vi "NATS Request.vi"(0 "nats connection in":T3={"connection ID"=refnum, "server INFO"="", "timeout ms"=5000, "verbose?"=FALSE, "server headers?"=FALSE, "client headers?"=FALSE}, 1 "reply-to":string, 2 "request queue":refnum<queue>, 5 "subject":string, 7 "payload":string, 9 "sub id":string, 11 "error in":errorcluster, 12 "timeout ms (conn default)":i32=-2, 13 "bytes to read (1024)":i32=1024) -> (4 "nats message":T1, 15 "error out":errorcluster)   [LabVIEW 2023, in "NATS Core.lvlib"]
doc: "Publishes a message to the NATS server."
uses:
  NATS Core.lvlib
  Controls/nats connection.ctl
  <vilib>/dlg_ctls.llb/Space Constant.vi
  subVIs/Set Timeout.vi
  Controls/msg type.ctl
  Controls/nats message.ctl
  Controls/request queue.ctl
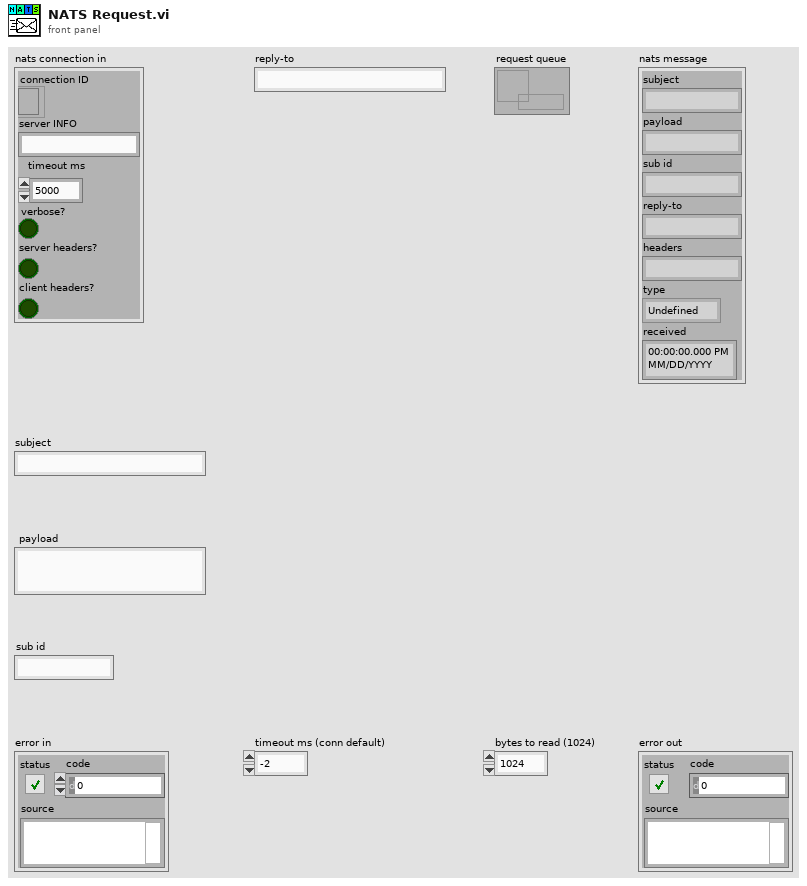
[diagram p1: front panel]
types:
  T1 = typedef "NATS Core.lvlib/nats message.ctl" = cluster{"subject":string, "payload":string, "sub id":string, "reply-to":string, "headers":string, "type":T2, "received":timestamp}
  T2 = typedef "NATS Core.lvlib/msg type.ctl" = enum16{"Undefined", "MSG", "HMSG", "+OK", "PING", "PONG", "-ERR", "INFO"}
  T3 = typedef "NATS Core.lvlib/nats connection.ctl" = cluster{"connection ID":refnum<k5>, "server INFO":string, "timeout ms":i32, "verbose?":bool, "server headers?":bool, "client headers?":bool}
  T4 = typedef "request queue.ctl" = cluster{"reply subject":string, "request queue":refnum<queue>}
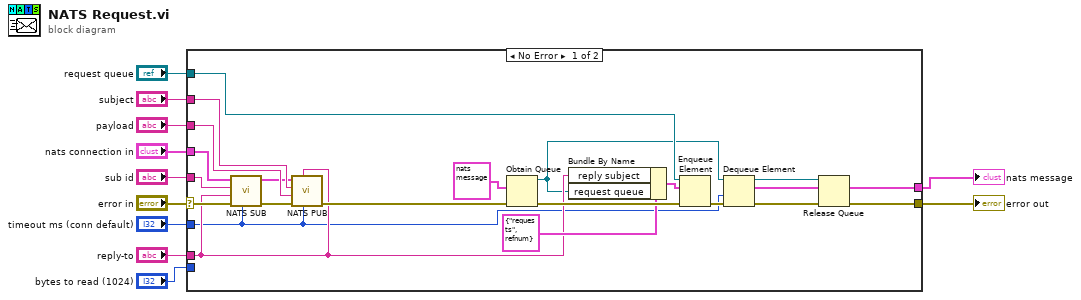
[diagram p0: block diagram]
diagram:
  n1 = case shown="No Error" "error in" {
    selector: "error in" -> [w32 w33]
    tunnel: "nats connection in" -> [w23 _]
    tunnel: "timeout ms (conn default)" -> [w15 _]
    tunnel: [w13 w33] -> w10
    tunnel: "subject" -> [w26 _]
    tunnel: "payload" -> [w25 _]
    tunnel: "reply-to" -> [w18 _]
    tunnel: "sub id" -> [w22 _]
    tunnel: "bytes to read (1024)" -> [_ _]
    tunnel: "request queue" -> [w20 _]
    tunnel: [w14 _] -> w1
    frame No Error {
      n2 = call "NATS SUB.vi"("timeout ms (conn default)"=w15, "error in"=w32, "subject"=w18, "sub id"=w22, "nats connection in"=w23) -> ("error out"=w31:errorcluster, "dup nats connection"=w24:T3)  [unwired: 4 in, 1 out]
      n3 = call "NATS PUB.vi"("timeout ms (conn default)"=w15, "reply-to"=w18, "error in"=w31, "payload"=w25, "subject"=w26, "nats connection in"=w24) -> ("error out"=w30:errorcluster)  [unwired: 4 in, 1 out]
      n4 = Obtain Queue(element data type=T1 {"subject"="", "payload"="", "sub id"="", "reply-to"="", "headers"="", "type"=enum."Undefined", "received"=timestamp(0 s since 1904-01-01)} ("nats message"), error in (no error)=w30) -> (queue out=w16:refnum<queue>, error out=w29:errorcluster)  [unwired: 3 in, 1 out]
      n5 = Bundle By Name(cluster=T4 {"reply subject"="requests", "request queue"=refnum} ("request queue"), "reply subject"=w18, "request queue"=w16) -> (w17:T4)
      n6 = Enqueue Element(queue=w20, element=w17, error in (no error)=w29) -> (error out=w28:errorcluster)  [unwired: 1 in, 2 out]
      n7 = Dequeue Element(queue=w16, timeout in ms (-1)=w15, error in (no error)=w28) -> (queue out=w12:refnum<queue>, element=w14:T1, error out=w27:errorcluster)  [unwired: 1 out]
      n8 = Release Queue(queue=w12, error in (no error)=w27) -> (error out=w13:errorcluster)  [unwired: 1 in, 2 out]
    }
    frame Error {
    }
  }
  "error out" <- w10
  "nats message" <- w1
